vi "Save position.vi"(2 "Position Graph":string, 3 "Position data":string, 5 "Step":dbl, 7 "Animal Number":dbl, 8 "RMS":dbl[][](array[numeric]), 9 "Normalized Position":dbl[][](array[numeric]), 10 "Position (output)":dbl[][](array[numeric]), 11 "Pos, Neg increments Position":dbl[][](array[numeric])) -> ()   [LabVIEW 2020]
panel:
  out "concatenated string 3":string
  out "concatenated string 2":string
  out "Position Waveforms":dbl[][](array[numeric])
  out "Position data":dbl[][](array[numeric])
  out "Position data":dbl[][](array[numeric])
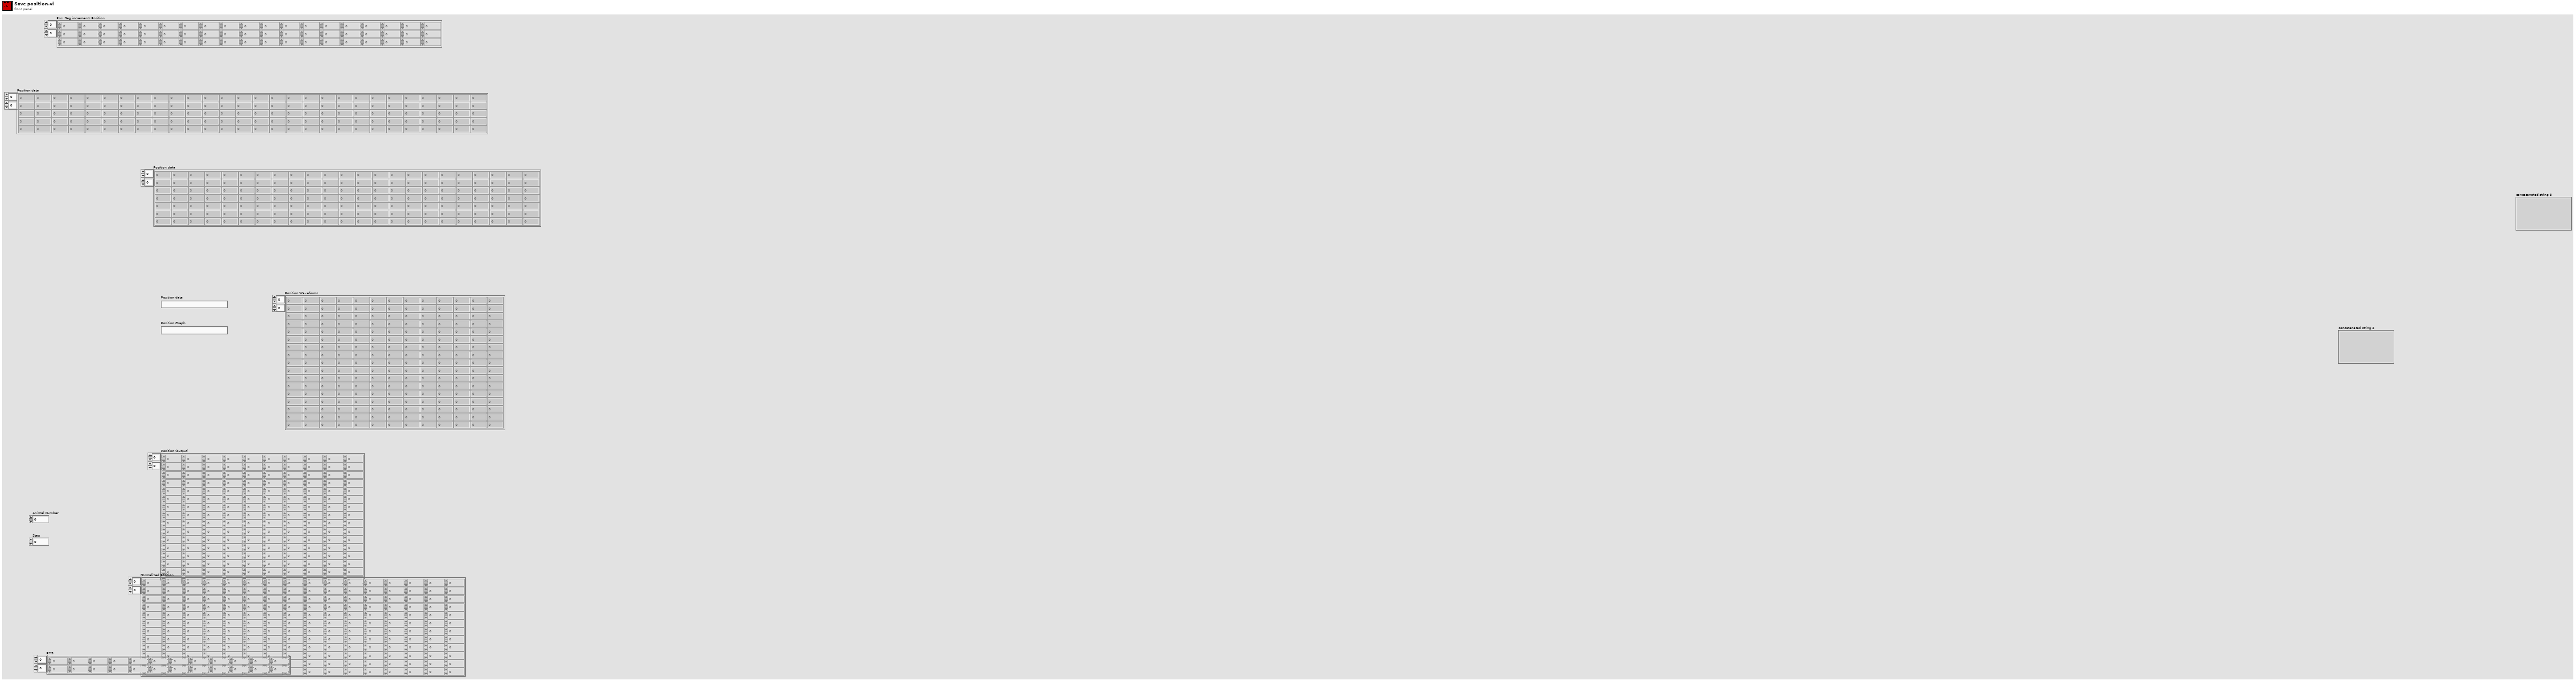
[diagram p1: front panel]
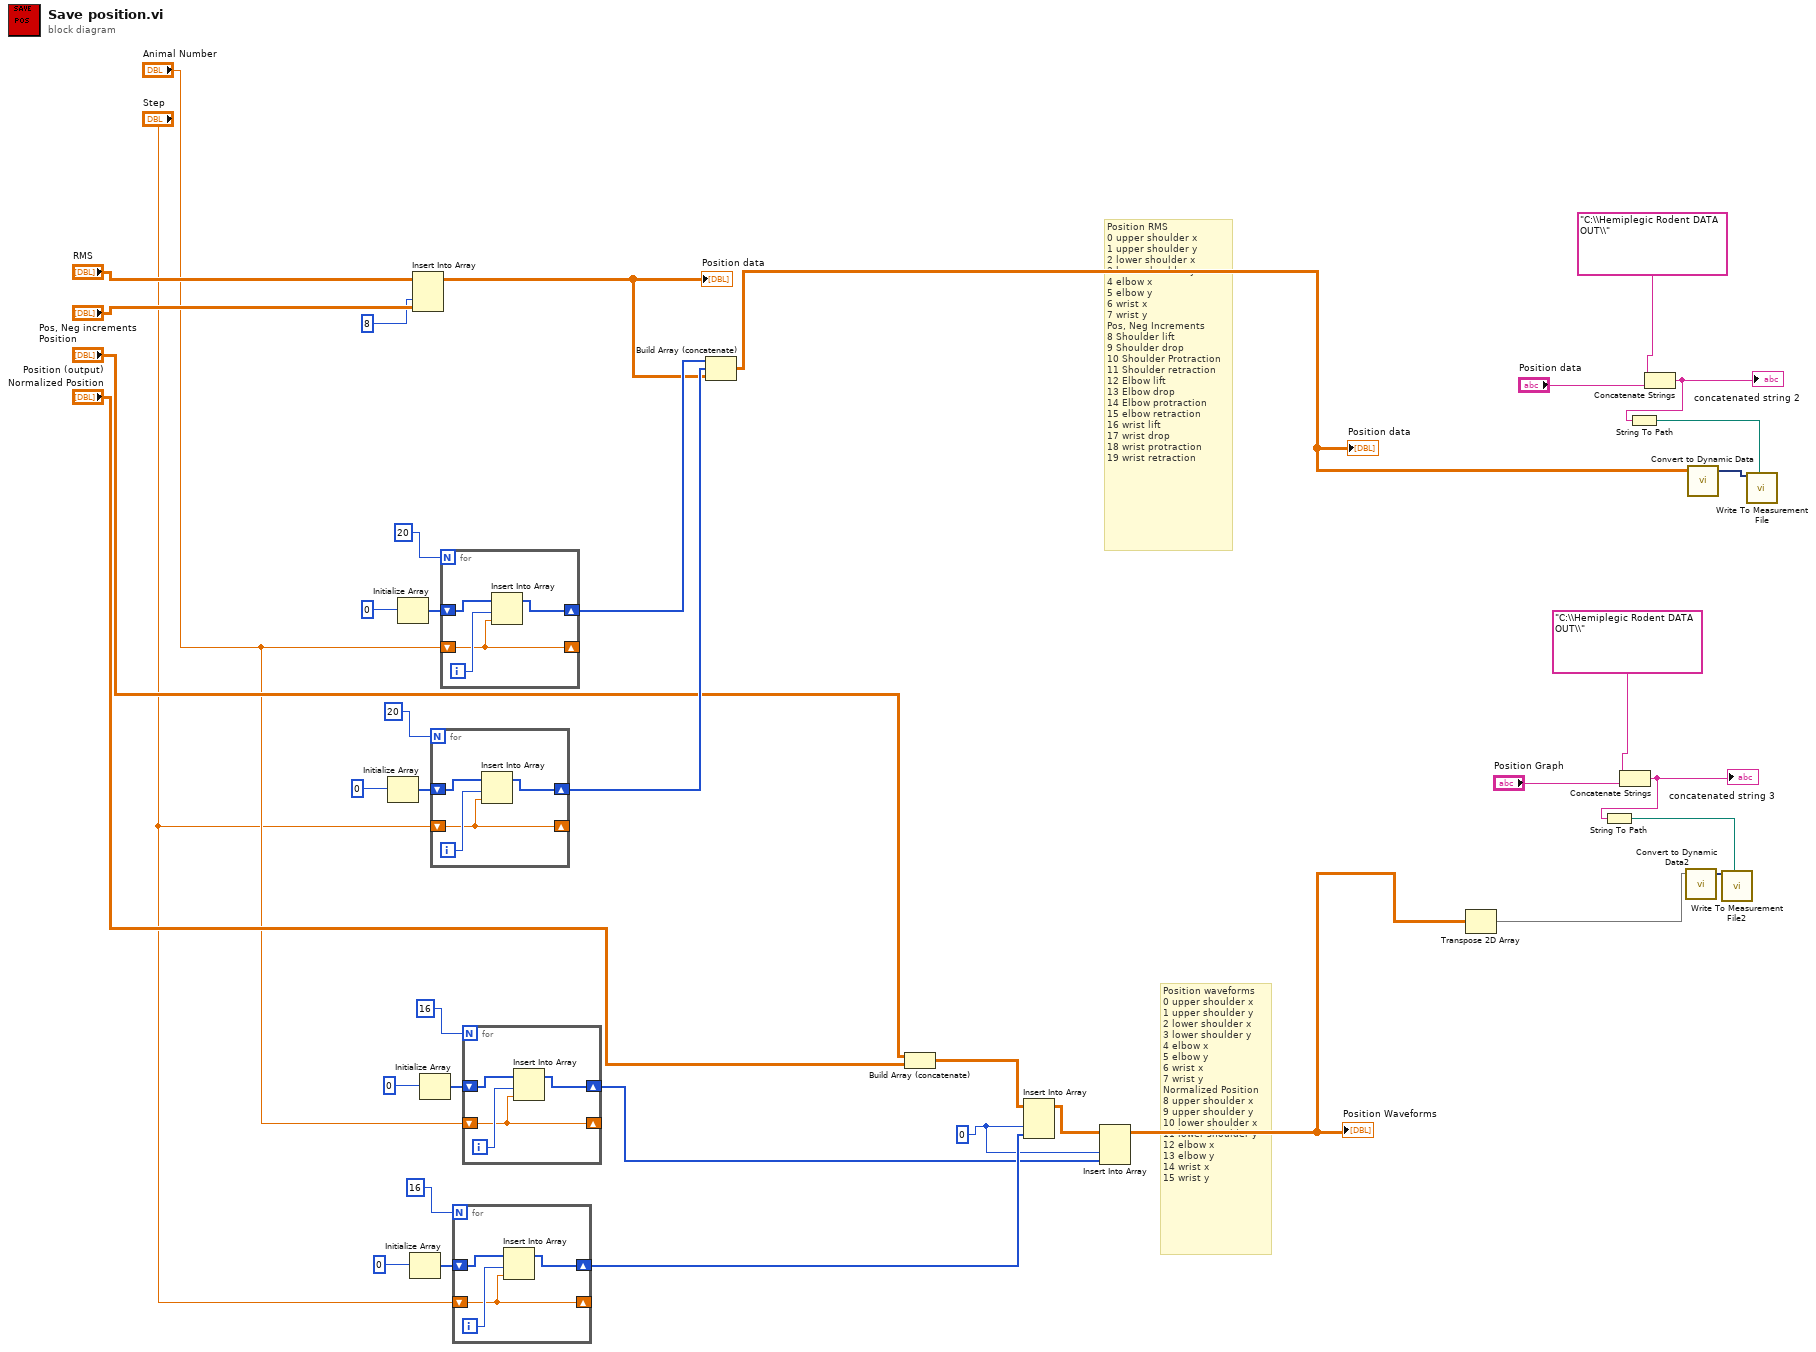
[diagram p0: block diagram]
diagram:
  w15 = 0
  # "Position waveforms\n0 upper shoulder x\n1 upper shoulder y\n2 lower shoulder x\n3 lower shoulder y\n4 elbow x\n5 elbow y\n6 wrist x\n7 wrist y\nNormalized Position\n8 upper shoulder x\n9 upper shoulder y\n10 lower shoulder x\n11 lower shoulder y\n12 elbow x\n13 elbow y\n14 wrist x\n15 wrist y"
  # "Position RMS\n0 upper shoulder x\n1 upper shoulder y\n2 lower shoulder x\n3 lower shoulder y\n4 elbow x\n5 elbow y\n6 wrist x\n7 wrist y\nPos, Neg Increments\n8 Shoulder lift\n9 Shoulder drop\n10 Shoulder Protraction\n11 Shoulder retraction\n12 Elbow lift\n13 Elbow drop\n14 Elbow protraction\n15 elbow retraction\n16 wrist lift\n17 wrist drop\n18 wrist protraction\n19 wrist retraction"
  n1 = Initialize Array(0) -> (w32:i32[])  [unwired: 1 in]
  n2 = Initialize Array(0) -> (w35:i32[])  [unwired: 1 in]
  n3 = Initialize Array(0) -> (w21:i32[])  [unwired: 1 in]
  n4 = Insert Into Array(array="RMS", index (col)=8, new element="Pos, Neg increments Position") -> (w29:dbl[][])  [unwired: 1 in]
  "Position data" <- w29
  n5 = Initialize Array(0) -> (w24:i32[])  [unwired: 1 in]
  n6 = for {
    N: 20 -> [_]
    shift-right: [w42] -> w30
    shift-left: w32 -> [w43]
    shift-right: [w41] -> _
    shift-left: "Step" -> [w41]
    i -> [w44]
    n7 = Insert Into Array(array=w43, index=w44, new element=w41) -> (w42:i32[])
  }
  n8 = for {
    N: 20 -> [_]
    shift-right: [w46] -> w31
    shift-left: w35 -> [w47]
    shift-right: [w45] -> _
    shift-left: "Animal Number" -> [w45]
    i -> [w48]
    n9 = Insert Into Array(array=w47, index=w48, new element=w45) -> (w46:i32[])
  }
  n10 = for {
    N: 16 -> [_]
    shift-right: [w50] -> w17
    shift-left: w21 -> [w51]
    shift-right: [w49] -> _
    shift-left: "Step" -> [w49]
    i -> [w52]
    n11 = Insert Into Array(array=w51, index=w52, new element=w49) -> (w50:i32[])
  }
  n12 = for {
    N: 16 -> [_]
    shift-right: [w54] -> w14
    shift-left: w24 -> [w55]
    shift-right: [w53] -> _
    shift-left: "Animal Number" -> [w53]
    i -> [w56]
    n13 = Insert Into Array(array=w55, index=w56, new element=w53) -> (w54:i32[])
  }
  n14 = Build Array (concatenate)(w31, w30, w29) -> (w9:dbl[][])
  "Position data" <- w9
  n15 = Build Array (concatenate)("Position (output)", "Normalized Position") -> (w18:dbl[][])
  n16 = Insert Into Array(array=w18, index (col)=w15, new element=w17) -> (w16:dbl[][])  [unwired: 1 in]
  n17 = Insert Into Array(array=w16, index (col)=w15, new element=w14) -> (w2:dbl[][])  [unwired: 1 in]
  "Position Waveforms" <- w2
  n18 = Transpose 2D Array(2D array=w2) -> (transposed array=w1:dbl[][])
  n19 = Concatenate Strings("C:\\Hemiplegic Rodent DATA OUT\\" ("name"), "Position Graph") -> (w6:string)
  "concatenated string 3" <- w6
  n20 = String To Path(string=w6) -> (path=w4:path)
  n21 = Concatenate Strings("C:\\Hemiplegic Rodent DATA OUT\\" ("name"), "Position data") -> (w12:string)
  "concatenated string 2" <- w12
  n22 = String To Path(string=w12) -> (path=w10:path)
  n23 = call "Convert to Dynamic Data2"("2D Array"=w1) -> ("Dynamic Data Type"=w3:dynamicdata)  [unwired: 3 in]
  n24 = call "Convert to Dynamic Data"("2D Array"=w9) -> ("Dynamic Data Type"=w8:dynamicdata)  [unwired: 3 in]
  n25 = call "Write To Measurement File2"("Signals"=w3, "Filename"=w4) -> ()  [unwired: 15 in, 3 out]
  n26 = call "Write To Measurement File"("Signals"=w8, "Filename"=w10) -> ()  [unwired: 15 in, 3 out]
